vi "set_new_position.vi"(8 "error in (no error)":errorcluster, 10 "set_pos":dbl[](array[numeric]), 11 "ESP301viaTCPIP in":refnum<class "ESP301viaTCPIP.lvclass">) -> (0 "error out":errorcluster, 3 "ESP301viaTCPIP out":refnum<class "ESP301viaTCPIP.lvclass">)   [LabVIEW 2019, in "ESP301viaTCPIP.lvlib" / "ESP301viaTCPIP.lvclass"]
uses:
  ESP301viaTCPIP.lvclass
  ESP301viaTCPIP.lvlib
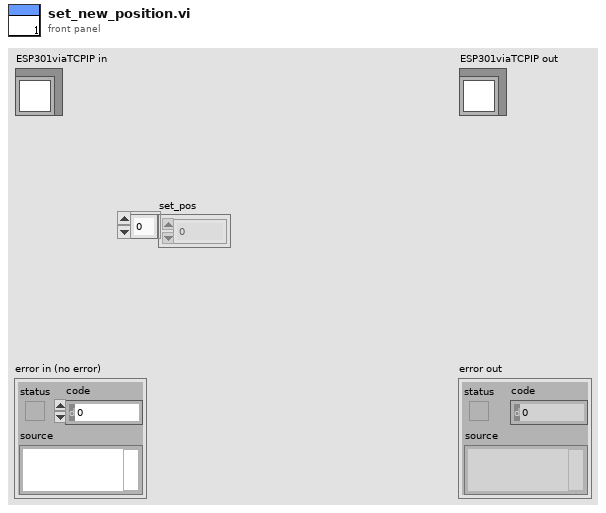
[diagram p1: front panel]
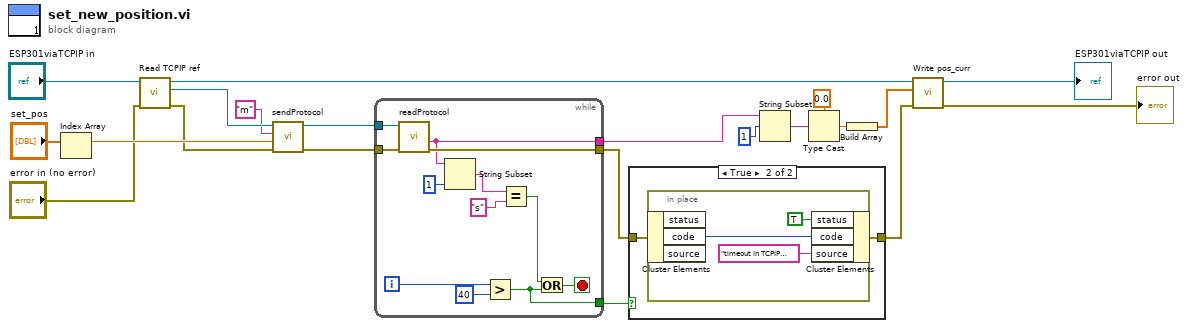
[diagram p0: block diagram]
diagram:
  n1 = Index Array(array="set_pos") -> (element=w18:dbl)  [unwired: 1 in]
  n2 = call-dynamic "Read TCPIP ref.vi"("error in (no error)"="error in (no error)", "ESP301viaTCPIP in"="ESP301viaTCPIP in") -> ("error out"=w16:errorcluster, "TCPIP ref"=w20:refnum<k5>, "ESP301viaTCPIP out"=w10:refnum<class "ESP301viaTCPIP.lvclass">)  [unwired: 7 in]
  n3 = call "sendProtocol.vi"("error in (no error)"=w16, "GoTo position"=w18, "command"="m", "TCP Network Connection in"=w20) -> ("error out"=w14:errorcluster, "TCP Network Connection out"=w15:refnum<k5>)  [unwired: 6 in]
  n4 = while {
    tunnel: w15 -> [w33]
    tunnel: w14 -> [w32]
    tunnel: [w28] -> w3
    tunnel: [w27] -> w13
    tunnel: [w22] -> w4
    i -> [w26]
    stop <- w23 stop-if-true
    n5 = call "readProtocol.vi"("error in (no error)"=w32, "TCP Network Connection in"=w33) -> ("error out"=w28:errorcluster, "data out"=w27:string)  [unwired: 8 in]
    n6 = String Subset(string=w27, length (rest)=1 ("length (rest)")) -> (substring=w30:string)  [unwired: 1 in]
    n7 = Greater?(x=w26, y=40) -> (0:w22:bool)
    n8 = Equal?(x=w30, y="s") -> (x = y?=w24:bool)
    n9 = Or(x=w24, y=w22) -> (x .or. y?=w23:bool)
  }
  n10 = case shown="True" w4 {
    tunnel: w3 -> [w34 w36]
    tunnel: [w34 w35] -> w2
    frame False {
    }
    frame True {
      n11 = in-place {
        n12 = in-place-cluster #1(w36) -> ("code"=w37:i32)  [unwired: 2 out]
        n13 = in-place-cluster #1("status"=TRUE, "code"=w37, "source"="timeout in TCPIP readback") -> (w35:errorcluster)
      }
    }
  }
  n14 = String Subset(string=w13, offset (0)=1 ("length (rest)")) -> (substring=w12:string)  [unwired: 1 in]
  n15 = Type Cast(type=0.0, x=w12) -> (*(type *) &x=w8:dbl)
  n16 = Build Array(w8) -> (w7:dbl[])
  n17 = call-dynamic "Write pos_curr.vi"("error in (no error)"=w2, "set_pos"=w7, "_stage in"=w10) -> ("error out"=→"error out":errorcluster, "_stage out"=→"ESP301viaTCPIP out":refnum<class "ESP301viaTCPIP.lvclass">)  [unwired: 7 in]
